vi "Stopwatch_Timer.vi"(0 "Start":bool, 5 "Pause":bool caption="Start", 9 "Reset":bool caption="Start", 11 "Stop":bool) -> (4 "hrs":i32, 6 "mins":i32, 8 "secs":i32, 10 "ms":dbl format="%#.3g")   [LabVIEW 2020]
doc: "This VI is a generic stopwatch timer which can be used for time calculations of the thinghs which are being done , By using this we can start, stop, pause, resume and reset the timer."
panel:
  in  "Resume":bool
  # "Stopwatch Timer"
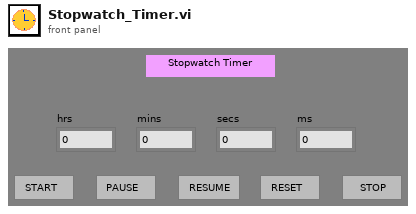
[diagram p1: front panel]
types:
  T1 = typedef "LVDateTimeRec.ctl" = cluster{"fractional second":dbl, "second":i32, "minute":i32, "hour":i32, "day of month":i32, "month":i32, "year":i32, "day of week":i32, "day of year":i32, "DST":i32}
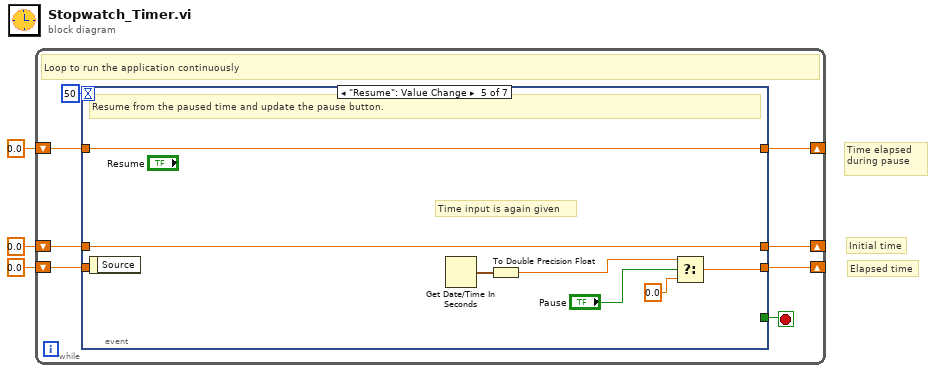
[diagram p0: block diagram]
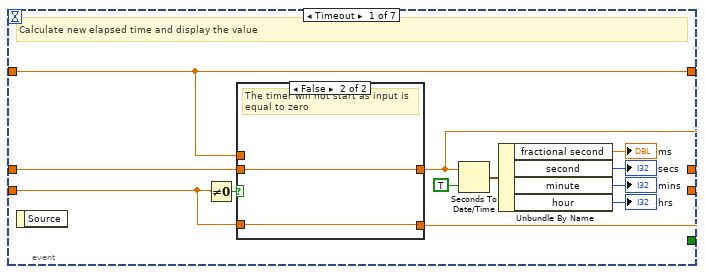
[diagram p2: hidden frame]
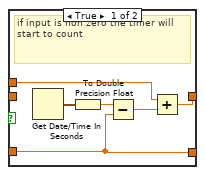
[diagram p3: hidden frame]
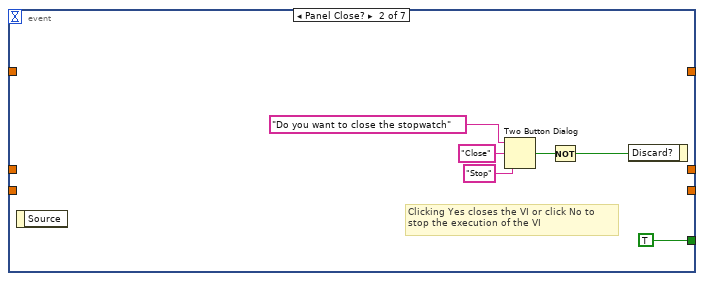
[diagram p4: hidden frame]
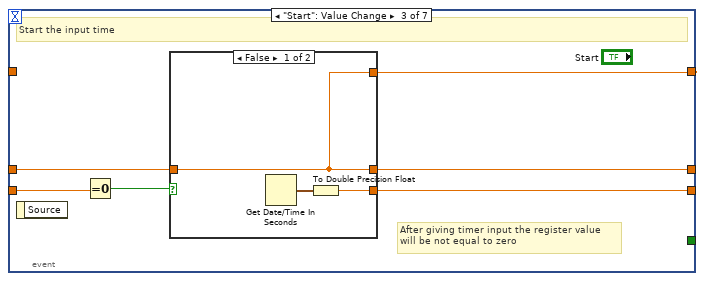
[diagram p5: hidden frame]
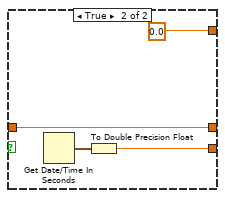
[diagram p6: hidden frame]
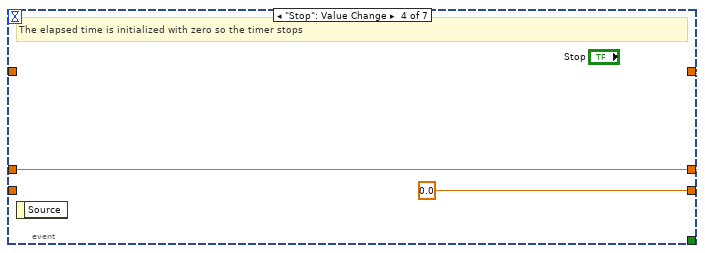
[diagram p7: hidden frame]
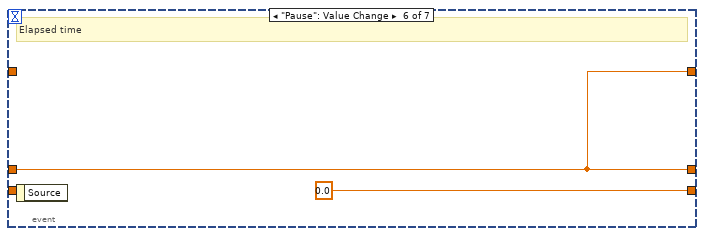
[diagram p8: hidden frame]
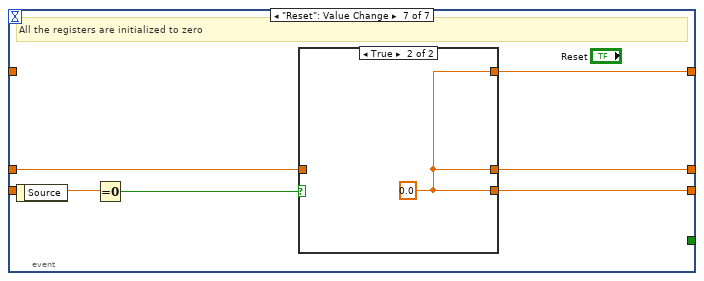
[diagram p9: hidden frame]
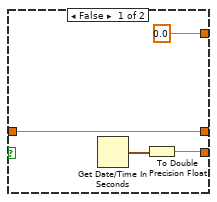
[diagram p10: hidden frame]
diagram:
  # "Time elapsed during pause"
  # "Elapsed time"
  # "Initial time"
  n1 = while {
    shift-right: [w7] -> _
    shift-left: 0.0 -> [w10]
    shift-right: [w8] -> _
    shift-left: 0.0 -> [w9]
    shift-right: [w5] -> _
    shift-left: 0.0 -> [w6]
    stop <- w4 stop-if-true
    # "Loop to run the application continuously"
    n2 = event shown="[4] \"Resume\": Value Change" {
      selector: _ -> [_ _ _ _ _ _ _]
      dyn-events: _ -> [_ _ _ _ _ _ _]
      timeout: 50 -> [_ _ _ _ _ _ _]
      tunnel: [w22 _ w43 0.0 w54 0.0 w63] -> w7
      tunnel: w10 -> [w12 _ w42 _ _ _ w67]
      tunnel: w9 -> [w23 _ w40 w52 w58 w60 w65]
      tunnel: [w16 _ w41 w52 w58 w60 w64] -> w8
      tunnel: [w15 _ w38 w52 w59 w60 w62] -> w5
      tunnel: w6 -> [w15 _ _ _ w59 _ _]
      tunnel: [_ TRUE _ _ _ _ _] -> w4
      event Timeout {
        # "Calculate new elapsed time and display the value"
        n3 = event-data() -> ()  [unwired: 1 in, 1 out]
        n4 = Not Equal To 0?(x=w12) -> (x != 0?=w13:bool)
        n5 = case shown="False" w13 {
          tunnel: w23 -> [_ w31]
          tunnel: [w24 w31] -> w16
          tunnel: w12 -> [w27 w30]
          tunnel: [w27 w30] -> w22
          tunnel: w15 -> [w25 _]
          frame True {
            # "if input is non zero the timer will start to count"
            n6 = Get Date/Time In Seconds() -> (seconds since 1Jan1904=w29:timestamp)
            n7 = To Double Precision Float(number=w29) -> (double precision float=w28:dbl)
            n8 = Subtract(x=w28, y=w27) -> (x-y=w26:dbl)
            n9 = Add(x=w25, y=w26) -> (x+y=w24:dbl)
          }
          frame False {
            # "The timer will not start as input is equal to zero"
          }
        }
        n10 = Seconds To Date/Time(time stamp (now)=w16, to UTC (F)=TRUE) -> (date time rec=w18:T1)
        n11 = Unbundle By Name(w18) -> ("fractional second"=→"ms":dbl, "second"=→"secs":i32, "minute"=→"mins":i32, "hour"=→"hrs":i32)
      }
      event Panel Close? {
        # "Clicking Yes closes the VI or click No to \nstop the execution of the VI"
        n12 = event-data() -> ()  [unwired: 1 in, 1 out]
        n13 = Two Button Dialog(message="Do you want to close the stopwatch", 1:"Stop" ("F button name (\"Cancel\")"), 2:"Close" ("T button name (\"OK\")")) -> (T button?=w35:bool)
        n14 = Not(x=w35) -> (.not. x?=w34:bool)
        n15 = event-data("Discard?"=w34) -> ()  [unwired: 1 in, 1 out]
      }
      event "Start": Value Change {
        # "After giving timer input the register value \nwill be not equal to zero"
        # "Start the input time"
        n16 = event-data() -> ()  [unwired: 1 in, 1 out]
        n17 = Equal To 0?(x=w42) -> (x = 0?=w39:bool)
        n18 = case shown="False" w39 {
          tunnel: [w45 w50] -> w43
          tunnel: [w44 w48] -> w41
          tunnel: w40 -> [w44 w48]
          tunnel: [w44 0.0] -> w38
          frame False {
            n19 = Get Date/Time In Seconds() -> (seconds since 1Jan1904=w46:timestamp)
            n20 = To Double Precision Float(number=w46) -> (double precision float=w45:dbl)
          }
          frame True {
            n21 = Get Date/Time In Seconds() -> (seconds since 1Jan1904=w49:timestamp)
            n22 = To Double Precision Float(number=w49) -> (double precision float=w50:dbl)
          }
        }
      }
      event "Stop": Value Change {
        # "The elapsed time is initialized with zero so the timer stops"
        n23 = event-data() -> ()  [unwired: 1 in, 1 out]
      }
      event "Resume": Value Change {
        # "Time input is again given"
        # "Resume from the paused time and update the pause button."
        n24 = event-data() -> ()  [unwired: 1 in, 1 out]
        n25 = Get Date/Time In Seconds() -> (seconds since 1Jan1904=w57:timestamp)
        n26 = To Double Precision Float(number=w57) -> (double precision float=w53:dbl)
        n27 = Select(t=w53, s="Pause", f=0.0) -> (s? t:f=w54:dbl)
      }
      event "Pause": Value Change {
        # "Elapsed time"
        n28 = event-data() -> ()  [unwired: 1 in, 1 out]
      }
      event "Reset": Value Change {
        # "All the registers are initialized to zero"
        n29 = event-data() -> ()  [unwired: 1 in, 1 out]
        n30 = Equal To 0?(x=w67) -> (x = 0?=w66:bool)
        n31 = case shown="True" w66 {
          tunnel: w65 -> [w70 _]
          tunnel: [w70 w72] -> w64
          tunnel: [w68 w72] -> w63
          tunnel: [0.0 w72] -> w62
          frame False {
            n32 = Get Date/Time In Seconds() -> (seconds since 1Jan1904=w69:timestamp)
            n33 = To Double Precision Float(number=w69) -> (double precision float=w68:dbl)
          }
          frame True {
            w72 = 0.0
          }
        }
      }
    }
  }
